vi "FlatSequenceStructures.vi"(7 "PythonConverter_BD in":refnum<class "PyConvBD.lvclass">, 8 "error in":errorcluster, 11 "Diagram in":refnum<class "Diagram.lvclass">) -> (0 "error out":errorcluster, 3 "Diagram out":refnum<class "Diagram.lvclass">, 4 "fss":string, 5 "PythonConverter_BD out":refnum<class "PyConvBD.lvclass">)   [LabVIEW 2014, in "Raspberry Pi Compatible Compiler for LabVIEW.lvlib" / "Diagram.lvclass"]
uses:
  Diagram.lvclass
  Python/PythonConverter_BD/PyConvBD.lvclass
  <vilib>/Utility/error.llb/whitespace.ctl
  Diagram.lvclass/Diagram.ctl
  FlatSequence/FlatSequence.lvclass/FlatSequence.ctl
  FlatSequence/FlatSequence.lvclass
  FlatSequenceFrame/FlatSequenceFrame.lvclass
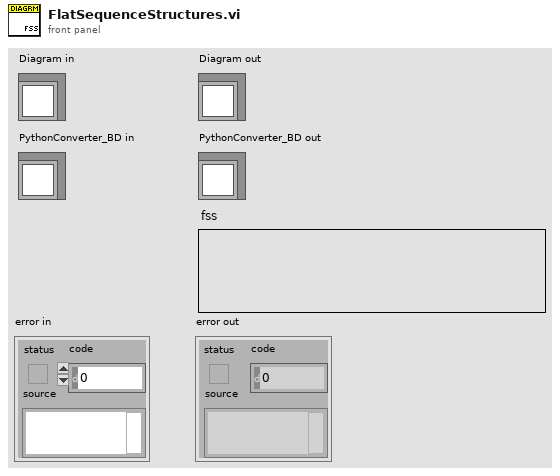
[diagram p1: front panel]
types:
  T1 = typedef "whitespace.ctl" = u16
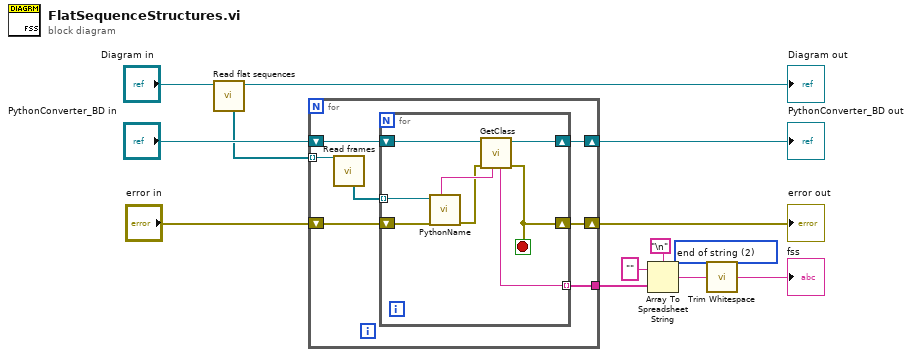
[diagram p0: block diagram]
diagram:
  w6 = T1 2 items=["both", "start of string", "end of string"] ("location (both)")
  n1 = call "Read flat sequences.vi"("Diagram in"="Diagram in") -> ("Diagram out"=→"Diagram out":refnum<class "Diagram.lvclass">, "flat sequences"=w2:refnum<class "FlatSequence.lvclass">[])  [unwired: 7 in]
  n2 = for {
    tunnel: w2 -> [w15] mode=indexing
    tunnel: [w16] -> w5
    shift-right: [w18] -> w11
    shift-left: "PythonConverter_BD in" -> [w20]
    shift-right: [w17] -> w10
    shift-left: "error in" -> [w19]
    n3 = call "Read frames.vi"("FlatSequence in"=w15) -> ("frames"=w14:refnum<class "FlatSequenceFrame.lvclass">[])  [unwired: 7 in, 1 out]
    n4 = for {
      tunnel: w14 -> [w25] mode=indexing
      shift-right: [w28] -> w18
      shift-left: w20 -> [w27]
      shift-right: [w22] -> w17
      shift-left: w19 -> [w26]
      tunnel: [w21] -> w16 mode=indexing
      stop <- w22 stop-if-true
      n5 = call-dynamic "PythonName.vi"("error in"=w26, "FlatSequenceFrame in"=w25) -> ("error out"=w23:errorcluster, "UID"=w24:string)  [unwired: 6 in, 2 out]
      n6 = call "GetClass.vi"("name"=w24, "error in"=w23, "PythonConverter_BD in"=w27) -> ("error out"=w22:errorcluster, "PythonConverter_BD out"=w28:refnum<class "PyConvBD.lvclass">, "class"=w21:string)  [unwired: 4 in]
    }
  }
  "error out" <- w10
  "PythonConverter_BD out" <- w11
  n7 = Array To Spreadsheet String(delimiter (Tab)="\n", array=w5, 3:"" ("format string")) -> (spreadsheet string=w7:string)
  n8 = call <vilib>:"Trim Whitespace.vi"("string"=w7, "location (both)"=w6) -> ("trimmed string"=→"fss":string)
